vi "Teleop.vi"(10 "Match Info":T1={"Autonomous Elapsed Seconds"=0.0, "TeleOp Elapsed Seconds"=0.0, "Disabled Elapsed Seconds"=0.0, "Visited Autonomous"=FALSE, "Visited TeleOp"=FALSE, "Visited Disabled"=FALSE, "Autonomous Settings"={"Autonomous Style"=enum."Independent", "VI Refnum"=refnum}}, 11 "Call Context":T2) -> ()   [LabVIEW 2011]
doc: "This VI is called for each TeleOp packet received from the DS where the robot is not disabled. It is often used to read from the joysticks and update I/O or to update setpoints for timed control loops. It should complete and return within 20 milliseconds or it may miss DS packets."
uses:
  <vilib>/Rock Robotics/WPI/DriverStation/WPI_DriverStationDerivedRobotMode.ctl
  <vilib>/Rock Robotics/WPI/DriverStation/WPI_DriverStationMatch Info.ctl
  Robot Global Data.vi
panel:
  out "Shift Control":dbl=2.0 format="%.2f"
  in  "Left High":dbl=0.2
  in  "Right High":dbl=0.8
  in  "Left Mid":dbl=0.25
  in  "Right Mid":dbl=0.7
  in  "Shift Input 2":dbl
  in  "Left Low":dbl=0.8
  in  "Right Low":dbl=0.4
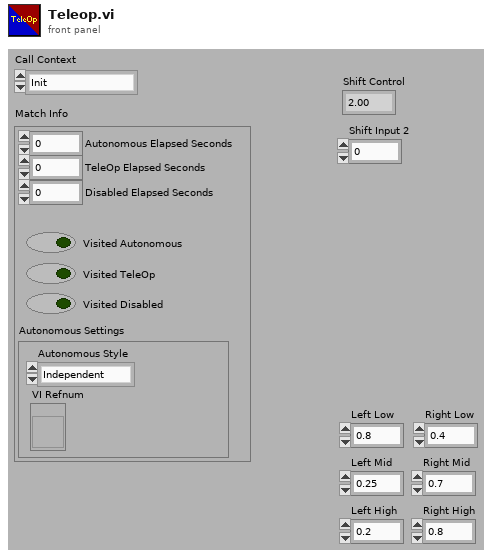
[diagram p1: front panel]
types:
  T1 = typedef "WPI_DriverStationMatch Info.ctl" = cluster{"Autonomous Elapsed Seconds":dbl, "TeleOp Elapsed Seconds":dbl, "Disabled Elapsed Seconds":dbl, "Visited Autonomous":bool, "Visited TeleOp":bool, "Visited Disabled":bool, "Autonomous Settings":cluster{"Autonomous Style":enum16{"Iterative", "Independent"}, "VI Refnum":refnum<vi>}}
  T2 = typedef "WPI_DriverStationDerivedRobotMode.ctl" = enum16{"Init", "Execute", "Stop"}
  T3 = typedef "WPI_JoystickDevRef.ctl" = cluster{"Device":T4}
  T4 = typedef "WPI_JoystickDeviceEnum.ctl" = enum16{"USB 1", "USB 2", "USB 3", "USB 4", "Kinect 1", "Kinect 2"}
  T5 = typedef "WPI_MotorControlDeviceRef.ctl" = cluster{"DeviceStatus":errorcluster, "Type":enum16{"PWM", "CAN"}, "PWM":cluster{"Digital Module":T6, "PWM Channel":T7, "DeadBand":T8}, "CAN":cluster{"Device Number":u8, "Control Mode":T9, "Semaphore":T10, "Max Vout":dbl}, "Invert":bool, "TransformRef":T11, "InvTransformRef":T11}
  T6 = typedef "FPGA_TypedefDigitalModule.ctl" = enum16{"Digital Module 1", "Digital Module 2"}
  T7 = typedef "FPGA_DIOPWMChannel.ctl" = enum8{"PWM 1", "PWM 2", "PWM 3", "PWM 4", "PWM 5", "PWM 6", "PWM 7", "PWM 8", "PWM 9", "PWM 10", "Invalid"}
  T8 = typedef "WPI_PWMDeadband.ctl" = cluster{"Name":string, "maxPositivePwm":i32, "minPositivePwm":i32, "centerPwm":i32, "maxNegativePwm":i32, "minNegativePwm":i32, "angularRange":u16}
  T9 = typedef "WPI_CANJaguar_ControlMode.ctl" = enum8{"Percent VBus", "Current", "Speed", "Position", "Voltage"}
  T10 = typedef "Semaphore RefNum" = refnum<k1>
  T11 = typedef "WPI_PWMTransform_ConPane.ctl" = refnum<vi>
  T12 = cluster{"axis 1 (x)":dbl, "axis 2 (y)":dbl, "axis 3 (throttle)":dbl, "axis 4":dbl, "axis 5":dbl, "axis 6":dbl}
  T13 = typedef "WPI_ServoDeviceRef.ctl" = cluster{"DeviceStatus":errorcluster, "Digital Module":T6, "PWM Channel":T7, "DeadBand":T8}
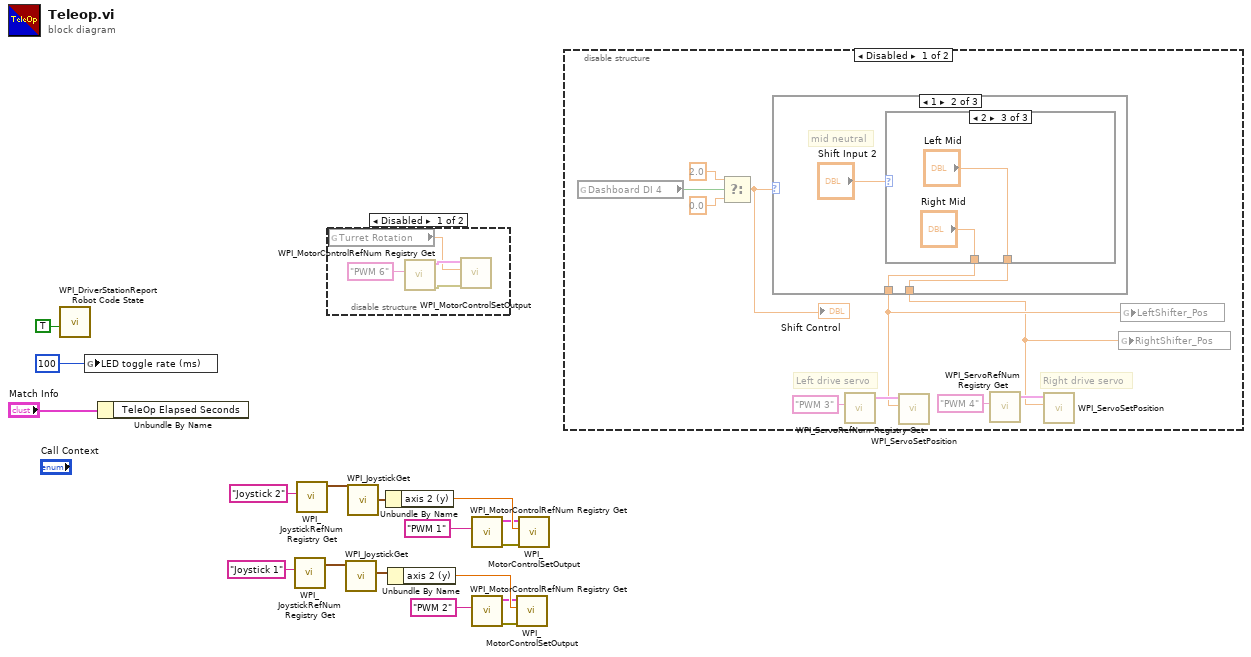
[diagram p0: block diagram]
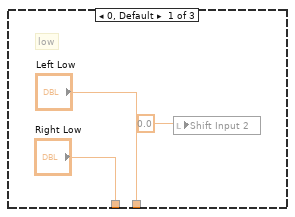
[diagram p2: hidden frame]
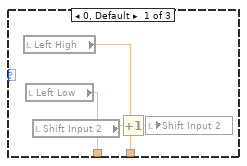
[diagram p3: hidden frame]
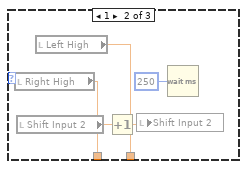
[diagram p4: hidden frame]
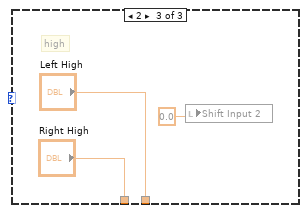
[diagram p5: hidden frame]
diagram:
  n1 = call <vilib>:"WPI_DriverStationReport Robot Code State.vi"("TeleOp"=TRUE ("Autonomous")) -> ()  [unwired: 10 in, 1 out]
  n2 = global write "Robot Global Data.vi" "LED toggle rate (ms)"(u32 100 ("LED ms toggle rate")) -> ()
  n3 = Unbundle By Name("Match Info") -> ()  [unwired: 1 out]
  n4 = call <vilib>:"WPI_JoystickRefNum Registry Get.vi"("refnum name"="Joystick 1") -> ("JoystickDevRef"=w7:T3)  [unwired: 9 in, 1 out]
  n5 = call <vilib>:"WPI_JoystickRefNum Registry Get.vi"("refnum name"="Joystick 2") -> ("JoystickDevRef"=w10:T3)  [unwired: 9 in, 1 out]
  n6 = disable-structure shown="Disabled" {
    frame Disabled {
      n7 = global read "Robot Global Data.vi" "Turret Rotation"() -> (w18:dbl)
      n8 = call <vilib>:"WPI_MotorControlRefNum Registry Get.vi"("refnum name"="PWM 6") -> ("error out"=w21:errorcluster, "MotorControlDevRef"=w20:T5)  [unwired: 9 in]
      n9 = call <vilib>:"WPI_MotorControlSetOutput.vi"("error in (no error)"=w21, "Output"=w18, "MotorControlDevRef"=w20) -> ()  [unwired: 7 in, 2 out]
    }
    frame Enabled {
    }
  }
  n10 = call <vilib>:"WPI_JoystickGet.vi"("JoystickDevRef"=w7) -> ("Axes"=w11:T12)  [unwired: 4 in, 2 out]
  n11 = call <vilib>:"WPI_JoystickGet.vi"("JoystickDevRef"=w10) -> ("Axes"=w14:T12)  [unwired: 4 in, 2 out]
  n12 = Unbundle By Name(w14) -> ("axis 2 (y)"=w12:dbl)
  n13 = Unbundle By Name(w11) -> ("axis 2 (y)"=w13:dbl)
  n14 = call <vilib>:"WPI_MotorControlRefNum Registry Get.vi"("refnum name"="PWM 1") -> ("error out"=w4:errorcluster, "MotorControlDevRef"=w3:T5)  [unwired: 9 in]
  n15 = call <vilib>:"WPI_MotorControlRefNum Registry Get.vi"("refnum name"="PWM 2") -> ("error out"=w6:errorcluster, "MotorControlDevRef"=w5:T5)  [unwired: 9 in]
  n16 = call <vilib>:"WPI_MotorControlSetOutput.vi"("error in (no error)"=w6, "Output"=w13, "MotorControlDevRef"=w5) -> ()  [unwired: 7 in, 2 out]
  n17 = call <vilib>:"WPI_MotorControlSetOutput.vi"("error in (no error)"=w4, "Output"=w12, "MotorControlDevRef"=w3) -> ()  [unwired: 7 in, 2 out]
  n18 = disable-structure shown="Disabled" {
    frame Disabled {
      # "Right drive servo"
      # "Left drive servo"
      n19 = global read "Robot Global Data.vi" "Dashboard DI 4"() -> (w24:bool)
      n20 = Select(t=2.0, s=w24, f=0.0) -> (s? t:f=w26:dbl)
      "Shift Control" <- w26
      n21 = case shown="1" w26 {
        tunnel: ["Left Low" w36 "Left High"] -> w22
        tunnel: ["Right Low" w35 "Right High"] -> w23
        frame 0, Default {
          # "low"
          n22 = local write "Shift Input 2"(0.0 ("Input 2")) -> ()
        }
        frame 1 {
          # "mid neutral"
          n23 = case shown="2" "Shift Input 2" {
            tunnel: [w41 w42 "Left Mid"] -> w36
            tunnel: [w40 w43 "Right Mid"] -> w35
            frame 0, Default {
              n24 = local read "Left High"() -> (w41:dbl)
              n25 = local read "Left Low"() -> (w40:dbl)
              n26 = local read "Shift Input 2"() -> (w39:dbl)
              n27 = Increment(x=w39) -> (x+1=w38:dbl)
              n28 = local write "Shift Input 2"(w38) -> ()
            }
            frame 1 {
              n29 = local read "Right High"() -> (w43:dbl)
              n30 = local read "Shift Input 2"() -> (w45:dbl)
              n31 = local read "Left High"() -> (w42:dbl)
              n32 = Increment(x=w45) -> (x+1=w44:dbl)
              n33 = local write "Shift Input 2"(w44) -> ()
              n34 = Wait (ms)(milliseconds to wait=u32 250) -> ()  [unwired: 1 out]
            }
            frame 2 {
            }
          }
        }
        frame 2 {
          # "high"
          n35 = local write "Shift Input 2"(0.0 ("Input 2")) -> ()
        }
      }
      n36 = call <vilib>:"WPI_ServoRefNum Registry Get.vi"("refnum name"="PWM 3") -> ("ServoDeviceRef"=w31:T13)  [unwired: 1 in, 9 out]
      n37 = call <vilib>:"WPI_ServoSetPosition.vi"("Position"=w23, "ServoDeviceRef"=w31) -> ()  [unwired: 1 in, 9 out]
      n38 = call <vilib>:"WPI_ServoRefNum Registry Get.vi"("refnum name"="PWM 4") -> ("ServoDeviceRef"=w27:T13)  [unwired: 1 in, 9 out]
      n39 = call <vilib>:"WPI_ServoSetPosition.vi"("Position"=w22, "ServoDeviceRef"=w27) -> ()  [unwired: 1 in, 9 out]
      n40 = global write "Robot Global Data.vi" "RightShifter_Pos"(w22) -> ()
      n41 = global write "Robot Global Data.vi" "LeftShifter_Pos"(w23) -> ()
    }
    frame Enabled {
    }
  }
